vi "Do.vi"(8 "error in (no error)":errorcluster, 10 "Actor in":refnum<class "Actor.lvclass">, 11 "Update Error Msg in":refnum<class "Update Error Msg.lvclass">) -> (0 "error out":errorcluster, 2 "Actor out":refnum<class "Actor.lvclass">)   [LabVIEW 2023, in "Example Iterator NR Actor Implicit Iteration.lvlib" / "Update Error Msg.lvclass"]
doc: "(<B>Filename</B>: Actor Framework.lvlib:Message.lvclass:Do.vi)\n\nDefines what a message does when it is received by an actor. Generally, a message instructs an actor to invoke one of its methods. By default, this method does nothing. A child class must override it to define behavior. Create a child class by using the Actor Framework Message Maker dialog box."
uses:
  Update Error Msg.lvclass
  C:/Projects/Iterator Actor/Iterator Actor/Iterator Actor Abstract Messages/Iterator Report Iterations End Msg/Iterator Report Iterations End Msg.lvclass
  <vilib>/ActorFramework/Actor/Actor.lvclass
  Example Actor/Example Actor.lvclass
  C:/Program Files/National Instruments/LabVIEW 2023/vi.lib/ActorFramework/Actor/Actor.lvclass
  Iterator Actor/Iterator Actor Abstract Messages/Iterator Report Iterations End Msg/Iterator Report Iterations End Msg.lvclass/Iterator Report Iterations End Msg.ctl
  Iterator Actor/Iterator Actor Abstract Messages/Iterator Report Iterations End Msg/Read Error 2.vi
  Iterator Actor/Iterator Actor Abstract Messages/Iterator Report Iterations End Msg/Read Stop Reason.vi
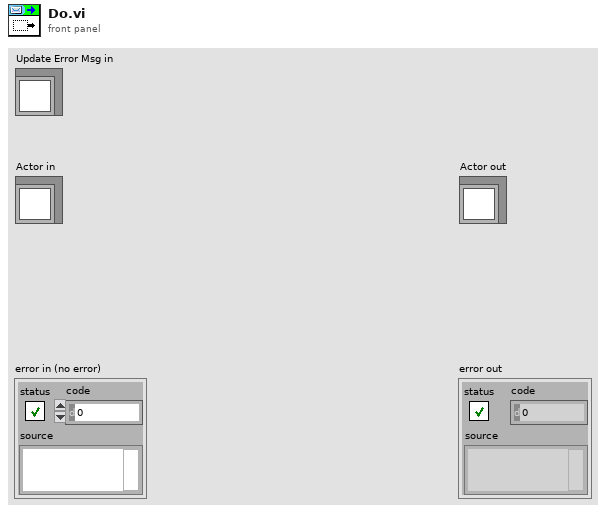
[diagram p1: front panel]
types:
  T1 = typedef "Iterator Actor.lvlib/Abstract Iterator Actor.lvclass/Stop Reason.ctl" = enum16{"Number of Iterations", "Time Elapsed", "Stopped Internally", "Stopped Externally"}
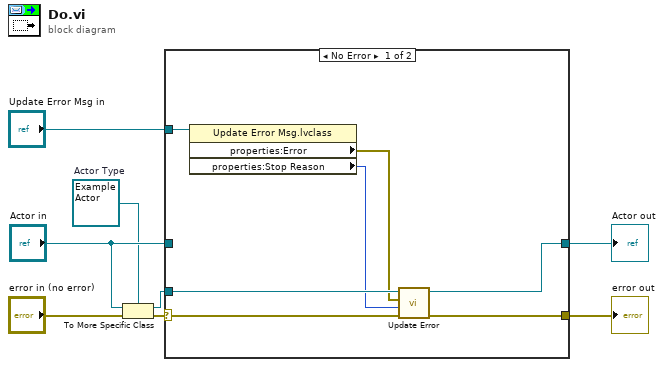
[diagram p0: block diagram]
diagram:
  w3 = refnum<class "Example Actor.lvclass"> refnum  # Actor Type
  n1 = To More Specific Class(target class=w3, reference="Actor in", error in="error in (no error)") -> (specific class reference=w2:refnum<class "Example Actor.lvclass">, error out=w7:errorcluster)
  n2 = case shown="No Error" w7 {
    selector: w7 -> [w13 w17]
    tunnel: [w15 w17] -> w6
    tunnel: [w14 w16] -> w5
    tunnel: "Actor in" -> [_ w16]
    tunnel: w2 -> [w12 _]
    tunnel: "Update Error Msg in" -> [w11 _]
    frame No Error {
      n3 = property class="Update Error Msg.lvclass"(reference=w11) -> ("properties:Error"=w10:errorcluster, "properties:Stop Reason"=w9:T1)  [unwired: 1 in, 2 out]
      n4 = call "Update Error.vi"("error in (no error)"=w13, "Stop Reason"=w9, "Received Error"=w10, "Example Actor in"=w12) -> ("error out"=w15:errorcluster, "Example Actor out"=w14:refnum<class "Example Actor.lvclass">)  [unwired: 6 in]
    }
    frame Error {
    }
  }
  "error out" <- w6
  "Actor out" <- w5
